vi "Module (Top Level).vi"(8 "error in":errorcluster) -> (0 "error out":errorcluster)   [LabVIEW 2017, in "myPAM.lvlib"]
uses:
  myPAM.lvlib
  MyPAM Controller/Controls/ControlVariables.ctl
  User Events/TypeDefs/Shutdown UE FGV Command.ctl
  Global TypeDefs/Registered Modules.ctl
  Public TypeDefs/Messages.ctl
  Public TypeDefs/Data for Logging.ctl
  MyPAM Controller/Controls/AdmittanceGains.ctl
  <vilib>/Platform/TimedLoop/XDataNode/timing_clust.ctl
  <vilib>/Platform/TimedLoop/XDataNode/nitl_modes.ctl
  <vilib>/Platform/TimedLoop/XDataNode/wakeup.ctl
  Libraries/Real time filter/TypeDefs/Modes.ctl
  Public TypeDefs/Current Position Data.ctl
  <vilib>/FPGAPlugInAG/myRIO-1900/niLvFpga_Open_myRIO-1900.vi
  <vilib>/Utility/error.llb/Error Cluster From Error Code.vi
  <vilib>/rvi/errors/niLvFpgaAdjustHostInterfaceError.vi
  <vilib>/FPGAPlugInAG/myRIO-1900/niLvFpga_Run_myRIO-1900.vi
  <vilib>/FPGAPlugInAG/myRIO-1900/niLvFpga_Close_myRIO-1900.vi
  <vilib>/rvi/interface/nirviOpenFPGA/nirviOpenFPGA.xnode
  <instrlib>/Devantech SRF02/FPGA Example/Serial/Private/FPGA Reference.ctl
  FPGA Bitfiles/myPAM_FPGATarget_FPGA(TopLevel)_Ff4lIePP4-I.lvbitx
  FPGA/FPGA (Top Level).vi
  <vilib>/rvi/interface/nirviReadWriteControl/nirviReadWriteControl.xnode
  <vilib>/rvi/interface/nirviMethod/nirviMethod.xnode
  <vilib>/Platform/TimedLoop/XDataNode/XDataNode.xnode
  <vilib>/rvi/interface/nirviCloseFPGA/nirviCloseFPGA.xnode
  Logger/Logger.lvlib
  Error Handler/Error Handler.lvlib
  Game/Game.lvlib
  <vilib>/Platform/TimedLoop/XDataNode/XDNodeRunTimeDep.lvlib
  WinHost/WinHost.lvlib
  Libraries/Real time filter/RealTimeFilter.lvlib
  NiFpgaLv.dll
  MyPAM Controller/controllerLibrary.lvlib
panel:
  in  "Tragety":dbl
  in  "Tragetx":dbl
  out "output cluster":T1={"ControlFlag"=TRUE, "Fx"=0.0, "Fy"=0.0, "Link1EncPos"=0.0, "Link2EncPos"=0.0, "CurrentX"=0.0, "CurrentY"=0.0, "TargetX"=0.0, "TargetY"=0.0, "DeadZone"=0.0}
  out "U2 2":dbl
  out "U1 2":dbl
  out "PID gains":T2
  out "U2":dbl
  out "U1":dbl
  out "?":cluster{dbl[], dbl[]}(graph)
  out "LINK1_Y_MM":fxp<+/-,34,16> format="%.23g"
  out "LINK1_X_MM":fxp<+/-,34,16> format="%.23g"
  out "LINK2_Y_MM":fxp<+/-,34,16> format="%.23g"
  out "LINK2_X_MM":fxp<+/-,34,16> format="%.23g"
  in  "Control flag":bool=TRUE
  out "LINK1_DEMAND":dbl
  out "LINK2_DEMAND":dbl
  # "mypam"
  # "game"
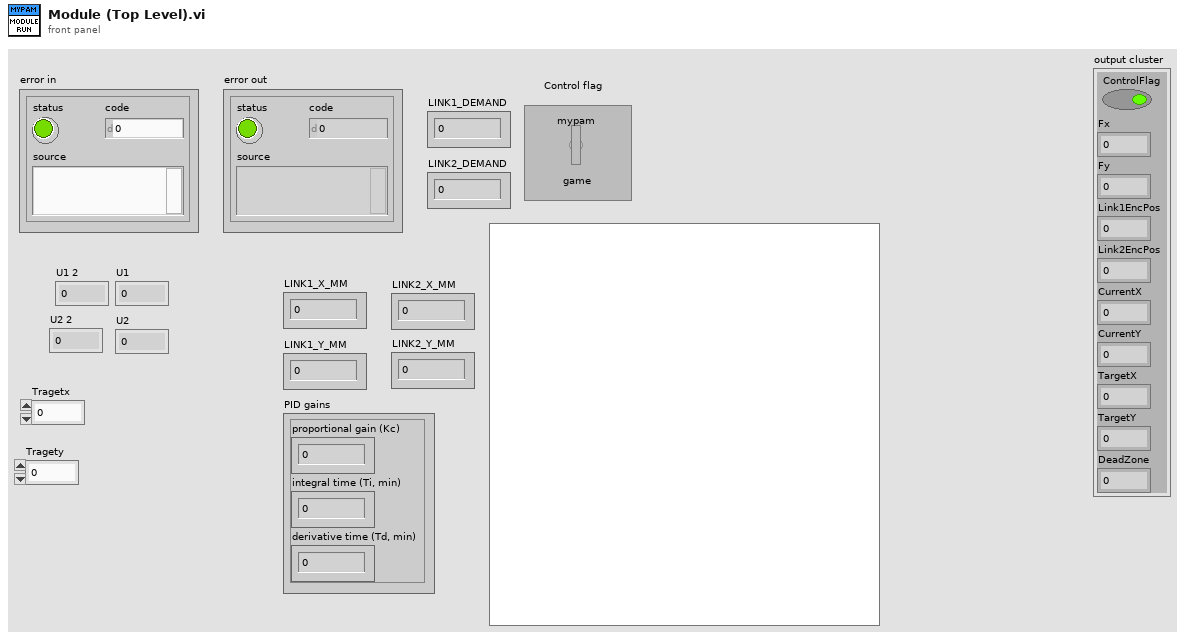
[diagram p1: front panel]
types:
  T1 = typedef "controllerLibrary.lvlib/ControlVariables.ctl" = cluster{"ControlFlag":bool, "Fx":dbl, "Fy":dbl, "Link1EncPos":dbl, "Link2EncPos":dbl, "CurrentX":dbl, "CurrentY":dbl, "TargetX":dbl, "TargetY":dbl, "DeadZone":dbl}
  T2 = cluster{"proportional gain (Kc)":dbl, "integral time (Ti, min)":dbl, "derivative time (Td, min)":dbl}
  T3 = typedef "Registered Modules.ctl" = enum16{"Controller", "DAQ", "Error Handler", "Game", "myPAM", "WinHost", "Logger"}
  T4 = typedef "Shutdown UE FGV Command.ctl" = enum16{"create", "get", "destroy"}
  T5 = typedef "WinHost.lvlib/Module Reference.ctl" = cluster{"calling module":T3, "module queues":T6, "module notifiers":T7}
  T6 = typedef "WinHost.lvlib/Module Queues.ctl" = cluster{"message queue":refnum<queue>, "STM queue":refnum<queue>}
  T7 = typedef "WinHost.lvlib/Module Notifiers.ctl" = cluster{"dummy notifier":refnum<notifier>}
  T8 = typedef "Game.lvlib/Module Reference.ctl" = cluster{"calling module":T3, "module queues":T9, "module notifiers":T10}
  T9 = typedef "Game.lvlib/Module Queues.ctl" = cluster{"message queue":refnum<queue>}
  T10 = typedef "Game.lvlib/Module Notifiers.ctl" = cluster{"dummy notifier":refnum<notifier>}
  T11 = typedef "Logger.lvlib/Module Reference.ctl" = cluster{"calling module":T3, "module queues":T12, "module notifiers":T13}
  T12 = typedef "Logger.lvlib/Module Queues.ctl" = cluster{"message queue":refnum<queue>}
  T13 = typedef "Logger.lvlib/Module Notifiers.ctl" = cluster{"dummy notifier":refnum<notifier>}
  T14 = typedef "myPAM.lvlib/Module Reference.ctl" = cluster{"calling module":T3, "module queues":T15, "module notifiers":T16}
  T15 = typedef "myPAM.lvlib/Module Queues.ctl" = cluster{"message queue":refnum<queue>}
  T16 = typedef "myPAM.lvlib/Module Notifiers.ctl" = cluster{"end eff. pos.":refnum<notifier>}
  T17 = typedef "Error Handler.lvlib/Module Reference.ctl" = cluster{"calling module":T3, "module queues":T18, "module notifiers":T19}
  T18 = typedef "Error Handler.lvlib/Module Queues.ctl" = cluster{"message queue":refnum<queue>}
  T19 = typedef "Error Handler.lvlib/Module Notifiers.ctl" = cluster{"dummy notifier":refnum<notifier>}
  T20 = cluster{"read mode":enum16{"polling", "blocking"}, "write mode":enum16{"polling", "blocking"}}
  T21 = typedef "myPAM.lvlib/Current Position Data.ctl" = cluster{"link 2 x (mm)":dbl, "link 2 y (mm)":dbl, "link 1 x (mm)":dbl, "link 1 y (mm)":dbl}
  T22 = typedef "XDNodeRunTimeDep.lvlib/timing_clust.ctl" = cluster{"Expected End [f-1]":u64, "Actual End [f-1]":u64, "Finished Late? [f-1]":bool, "Expected End [i-1]":u64, "Actual End [i-1]":u64, "Finished Late? [i-1]":bool, "Expected Start [i]":u64, "Actual Start [i]":u64, "Expected Start [f]":u64, "Actual Start [f]":u64, "Source Name":string, "Structure Name":string, "Period":i64, "Deadline":i64, "Offset":i64, "Start":i64, "Priority":i32, "Timeout":i32, "Mode":T23, "Wakeup Reason":T24, "Error":errorcluster, "Source Type":string, "Secondary Source Type":string, "Global End Time":u64, "Global Start Time":u64, "Frame Duration":u64, "Iteration Duration":u64, "Assigned CPU":i32, "I/O Scan Engine Mode":u32}
  T23 = typedef "XDNodeRunTimeDep.lvlib/nitl_modes.ctl" = enum32{"No Change", "Process missed periods, maintain original phase", "Discard missed periods, maintain original phase", "Process missed periods, ignore original phase", "Discard missed periods, ignore original phase"}
  T24 = typedef "XDNodeRunTimeDep.lvlib/wakeup.ctl" = enum32{"Normal", "Aborted", "Asynchronous wakeup", "Timing source error", "Timed loop error", "Timeout"}
  T25 = typedef "FPGA Reference.ctl" = refnum<k20>
  T26 = typedef "myPAM.lvlib/Messages.ctl" = enum16{"calibrate encoders", "enable motors", "disable motors", "operate", "shutdown"}
  T27 = typedef "controllerLibrary.lvlib/AdmittanceGains.ctl" = cluster{"C":dbl, "k":dbl}
  T28 = typedef "myPAM.lvlib/Data for Logging.ctl" = cluster{"end effector x (mm)":dbl, "end effector y (mm)":dbl, "target x (mm)":dbl, "target y (mm)":dbl, "Theta 1":dbl, "Theta 2":dbl, "Omega 1":dbl, "Omega 2":dbl}
  T29 = typedef "myPAM.lvlib/RealTimeFilter.lvlib/Parameters.ctl" = cluster{"number of elements":i32, "start value":dbl, "sinusoidal profile":dbl[], "gaussian profile":dbl[]}
  T30 = typedef "myPAM.lvlib/RealTimeFilter.lvlib/Modes.ctl" = enum16{"Sinusoidal", "Gaussian"}
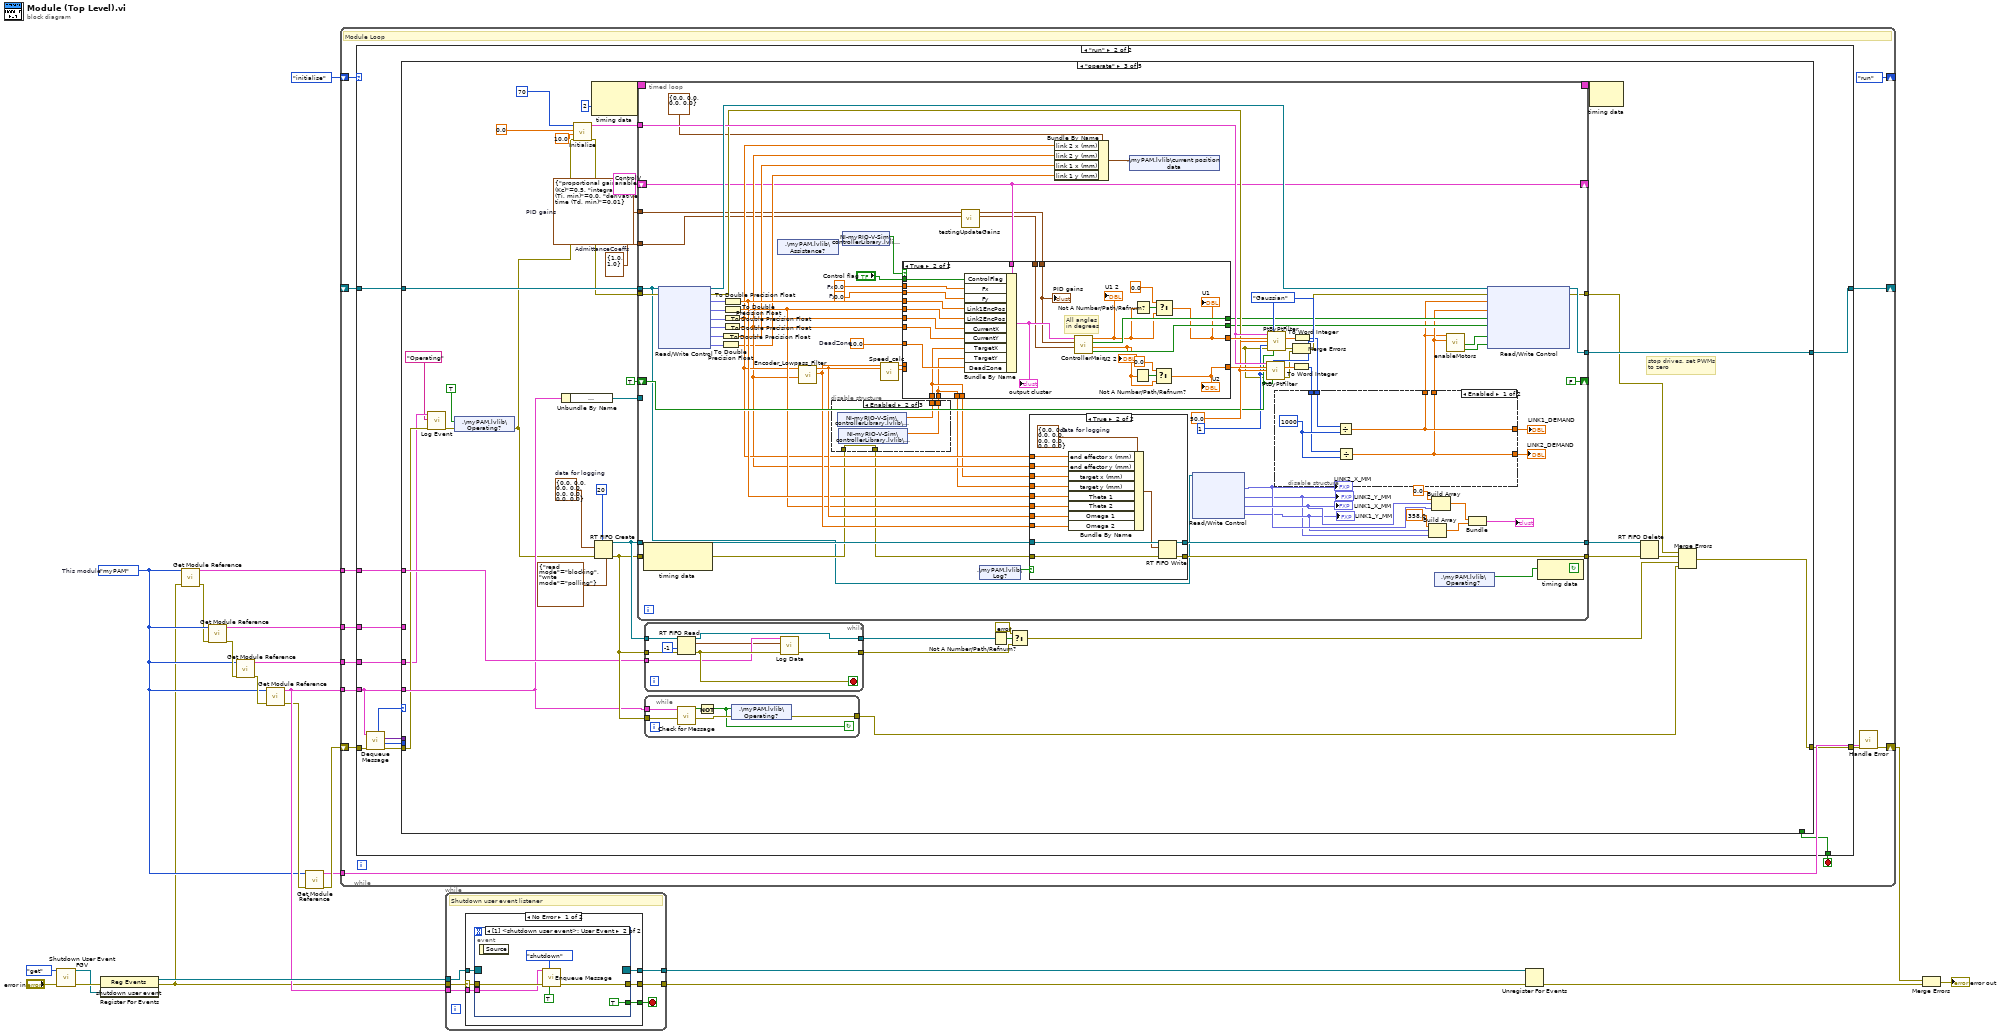
[diagram p0: block diagram]
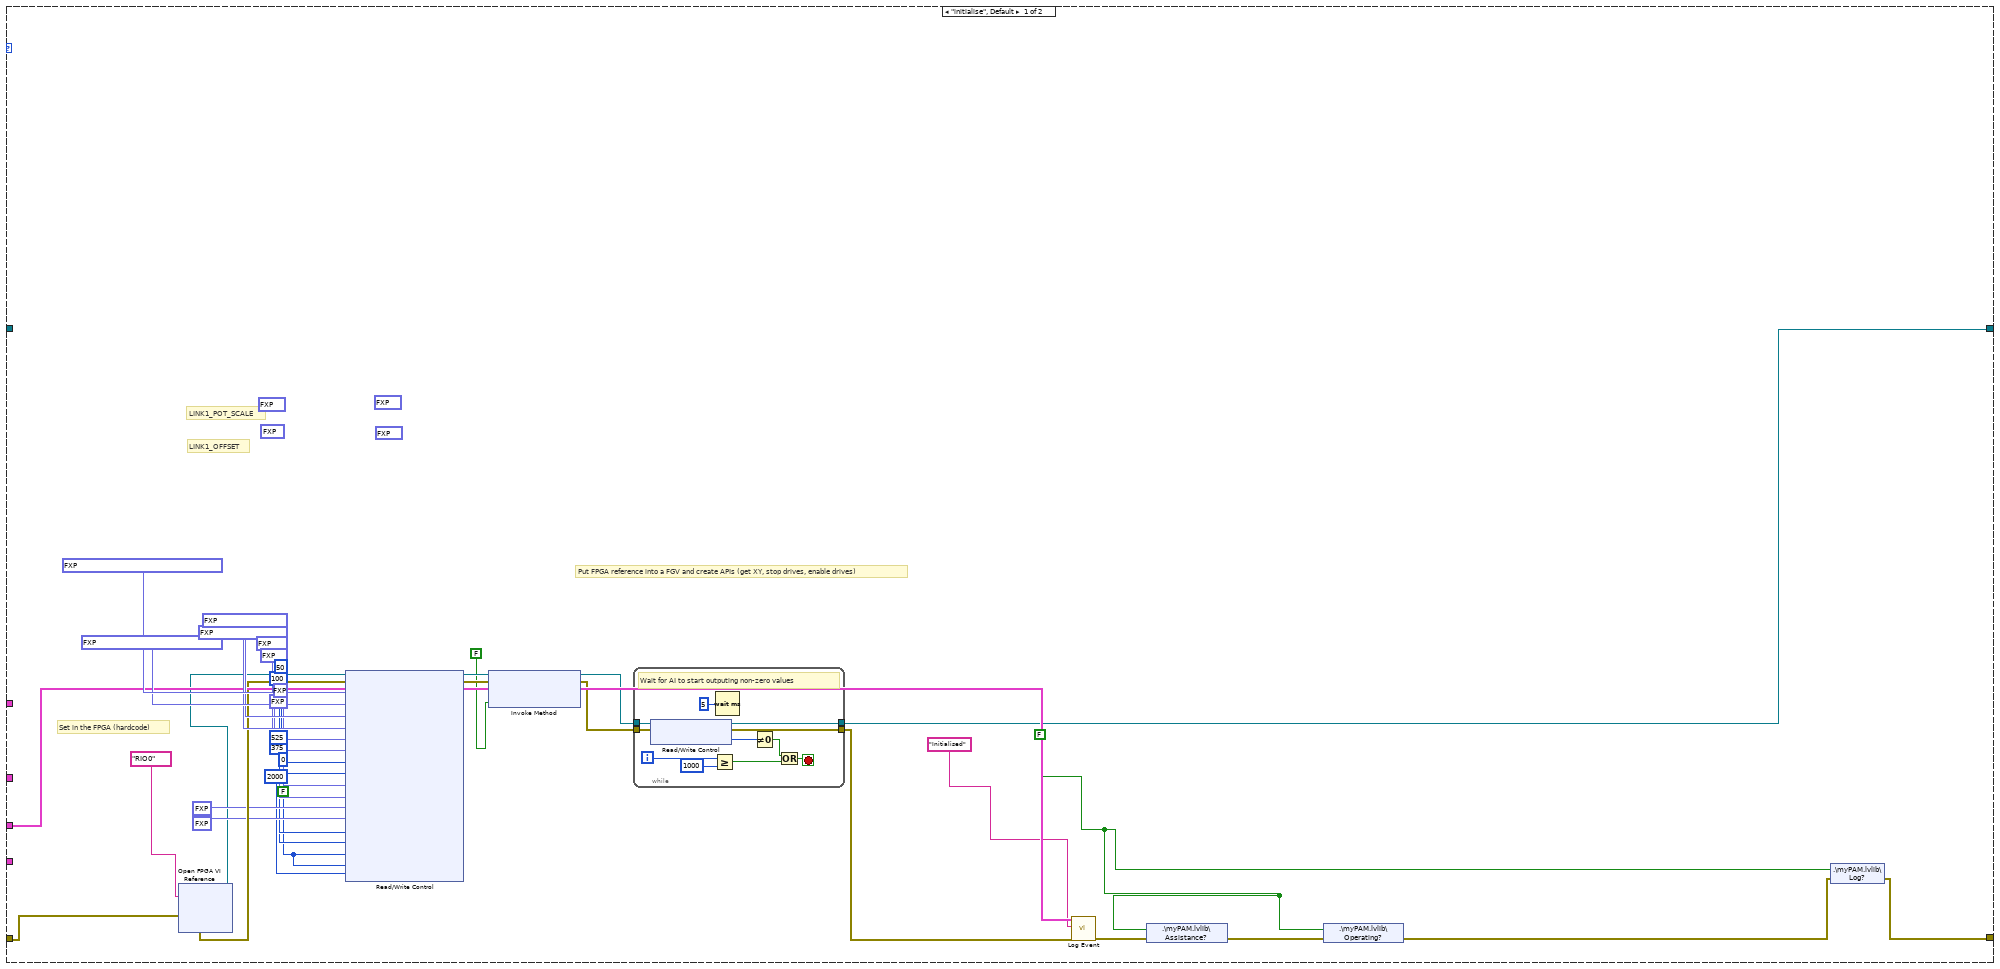
[diagram p2: hidden frame]
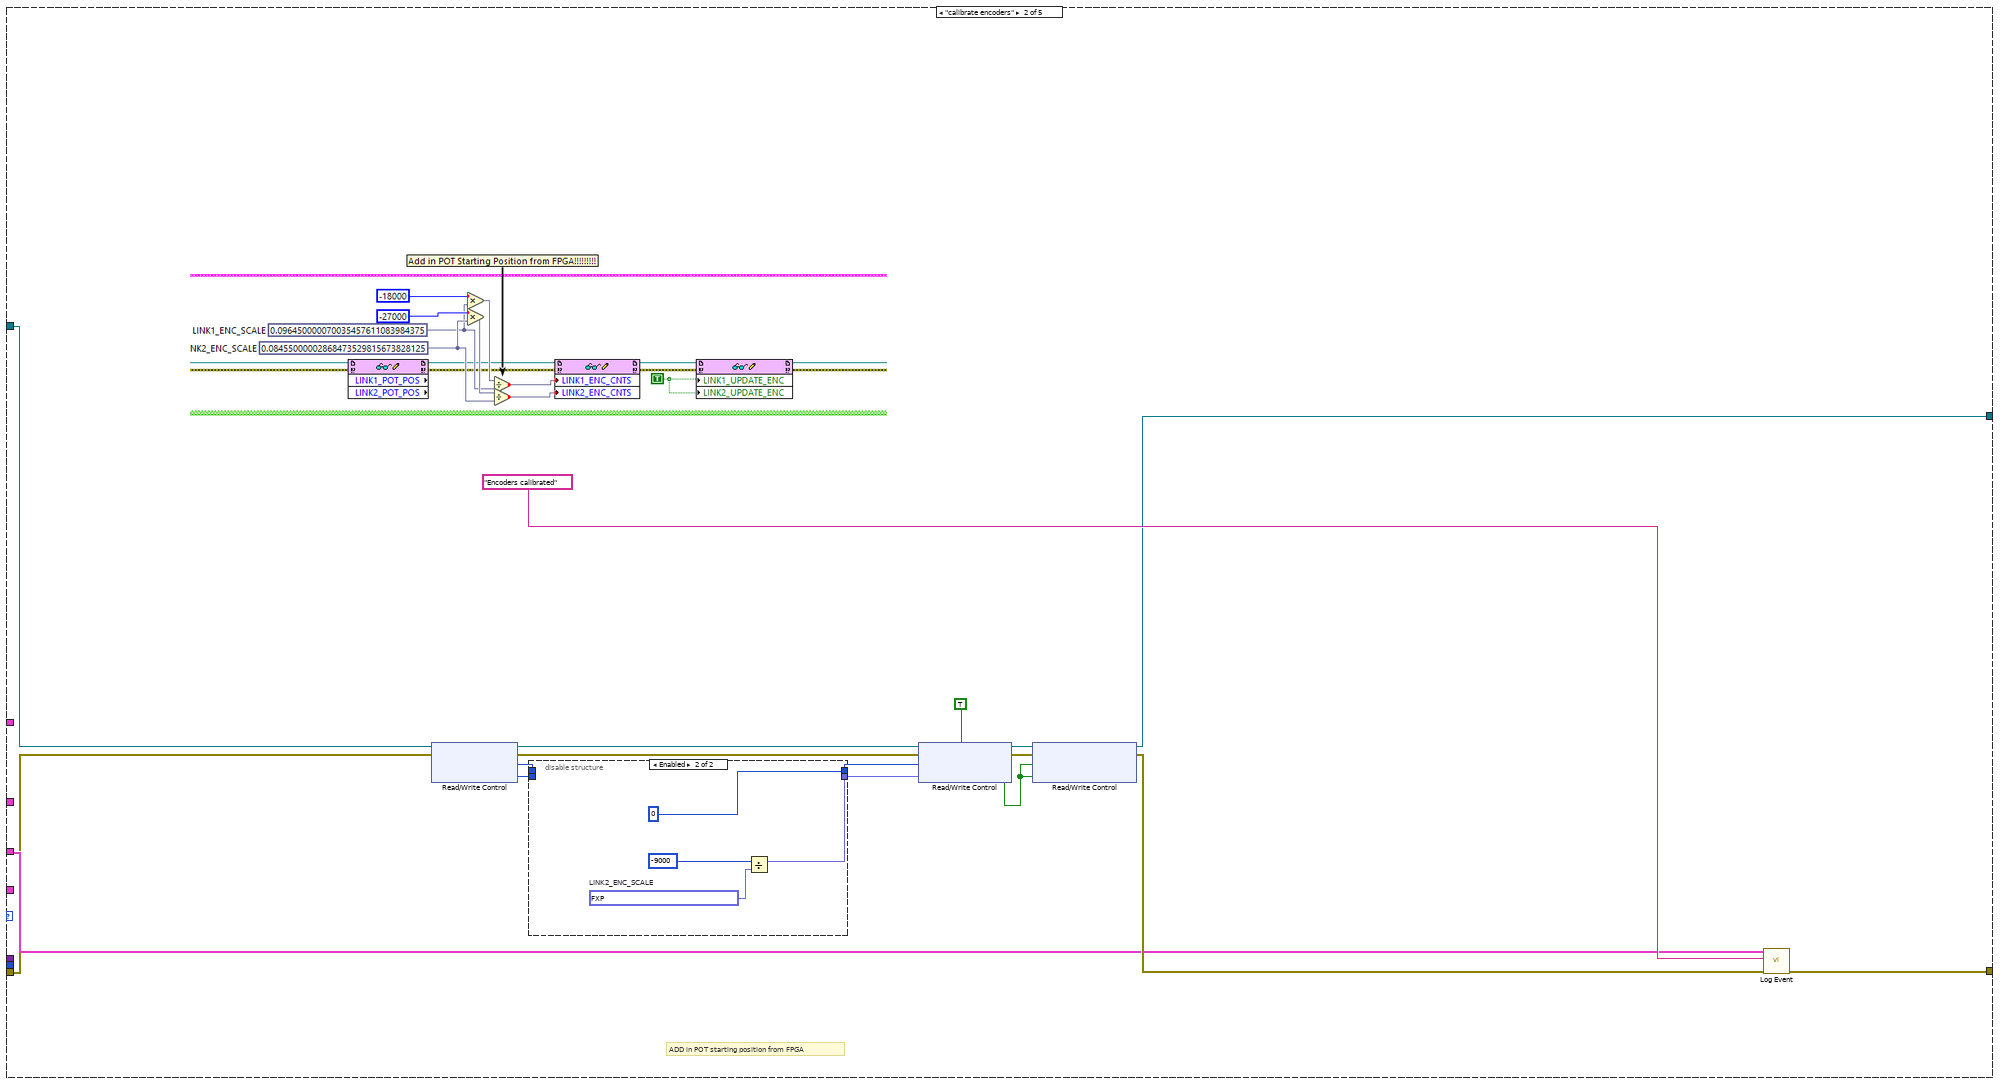
[diagram p4: hidden frame]
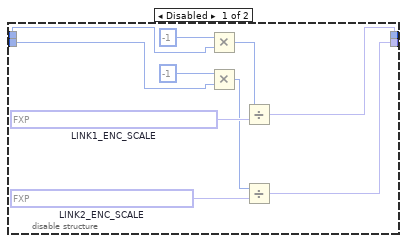
[diagram p5: hidden frame]
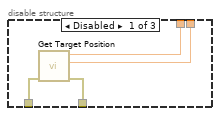
[diagram p6: hidden frame]
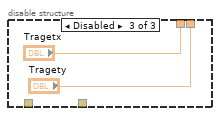
[diagram p7: hidden frame]
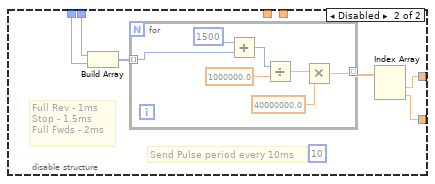
[diagram p8: hidden frame]
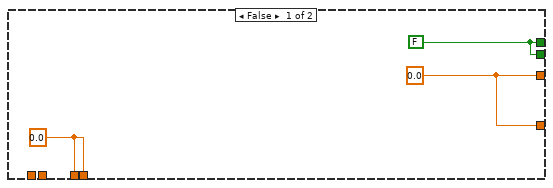
[diagram p9: hidden frame]
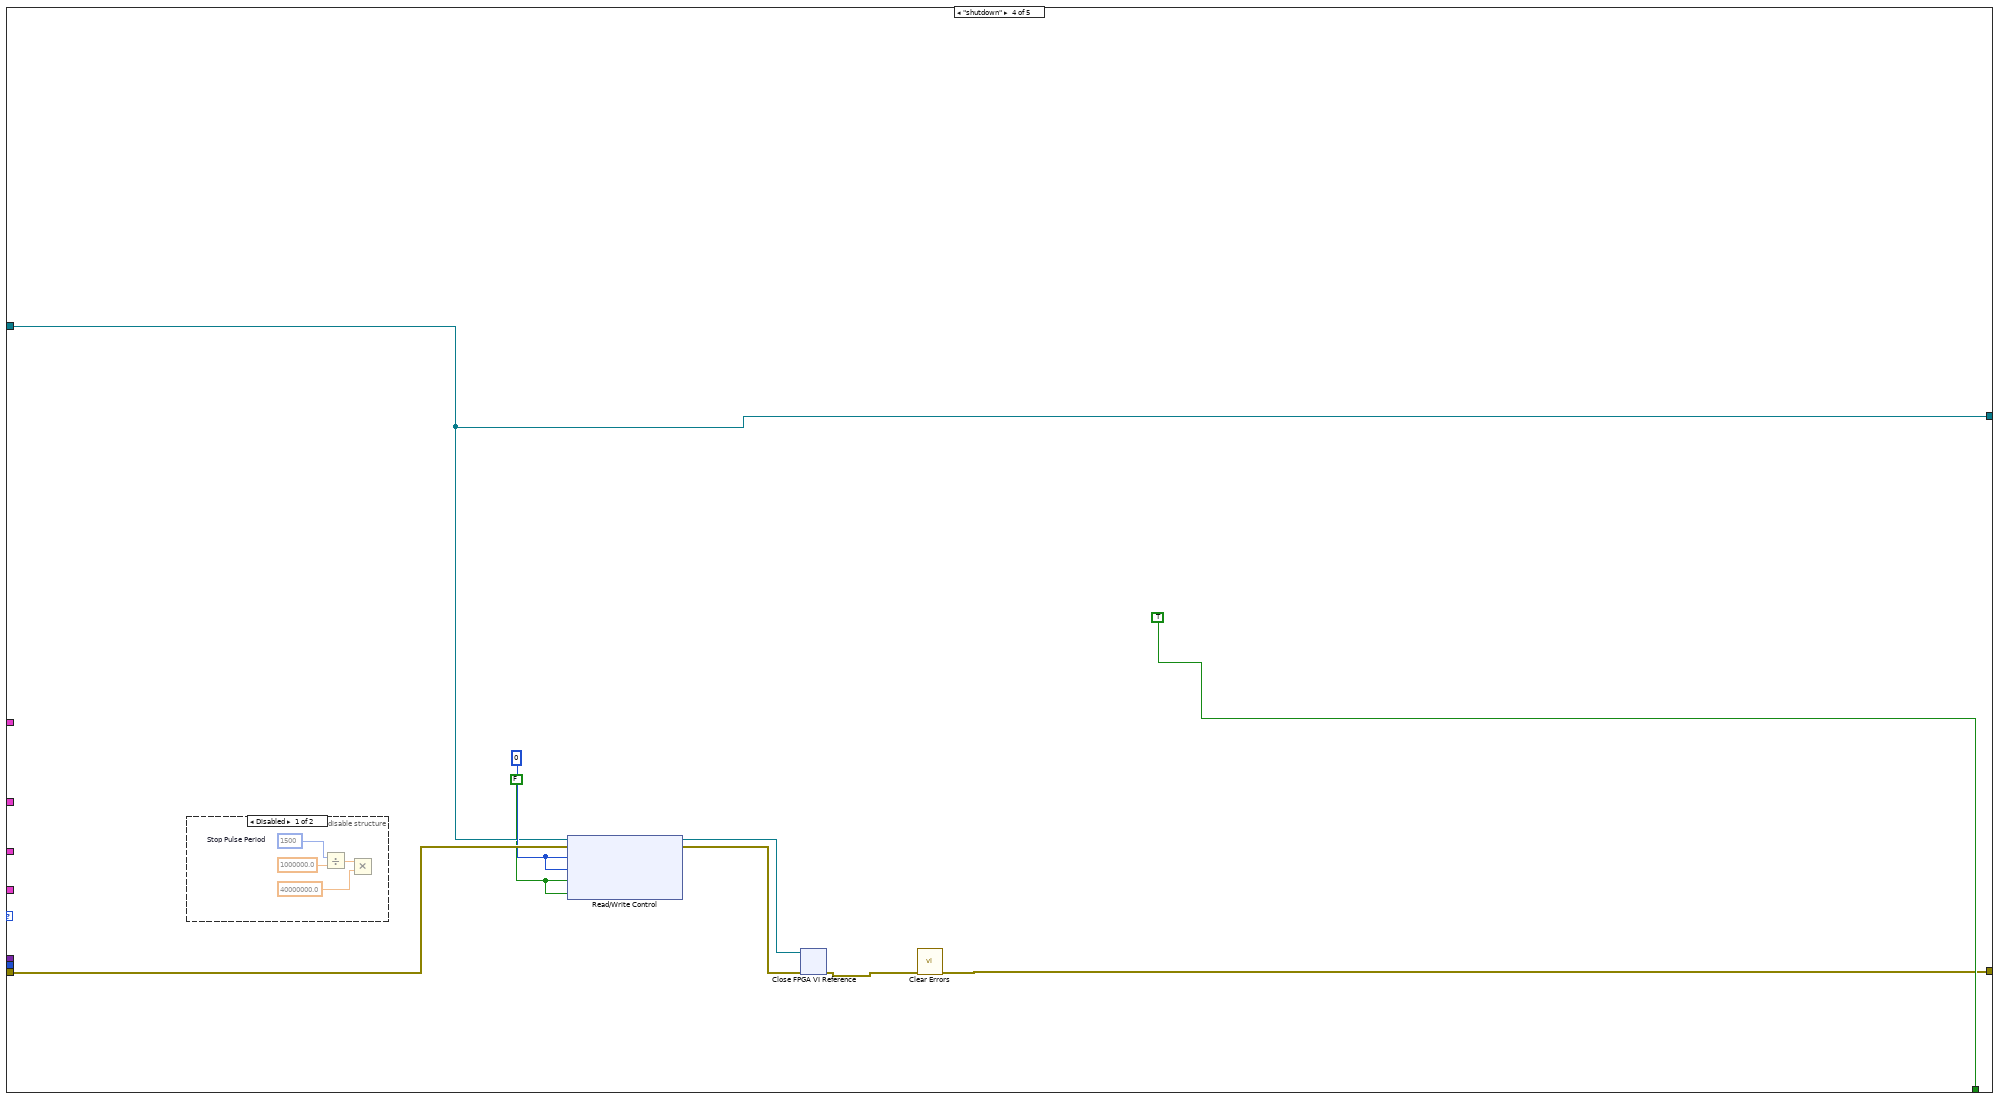
[diagram p11: hidden frame]
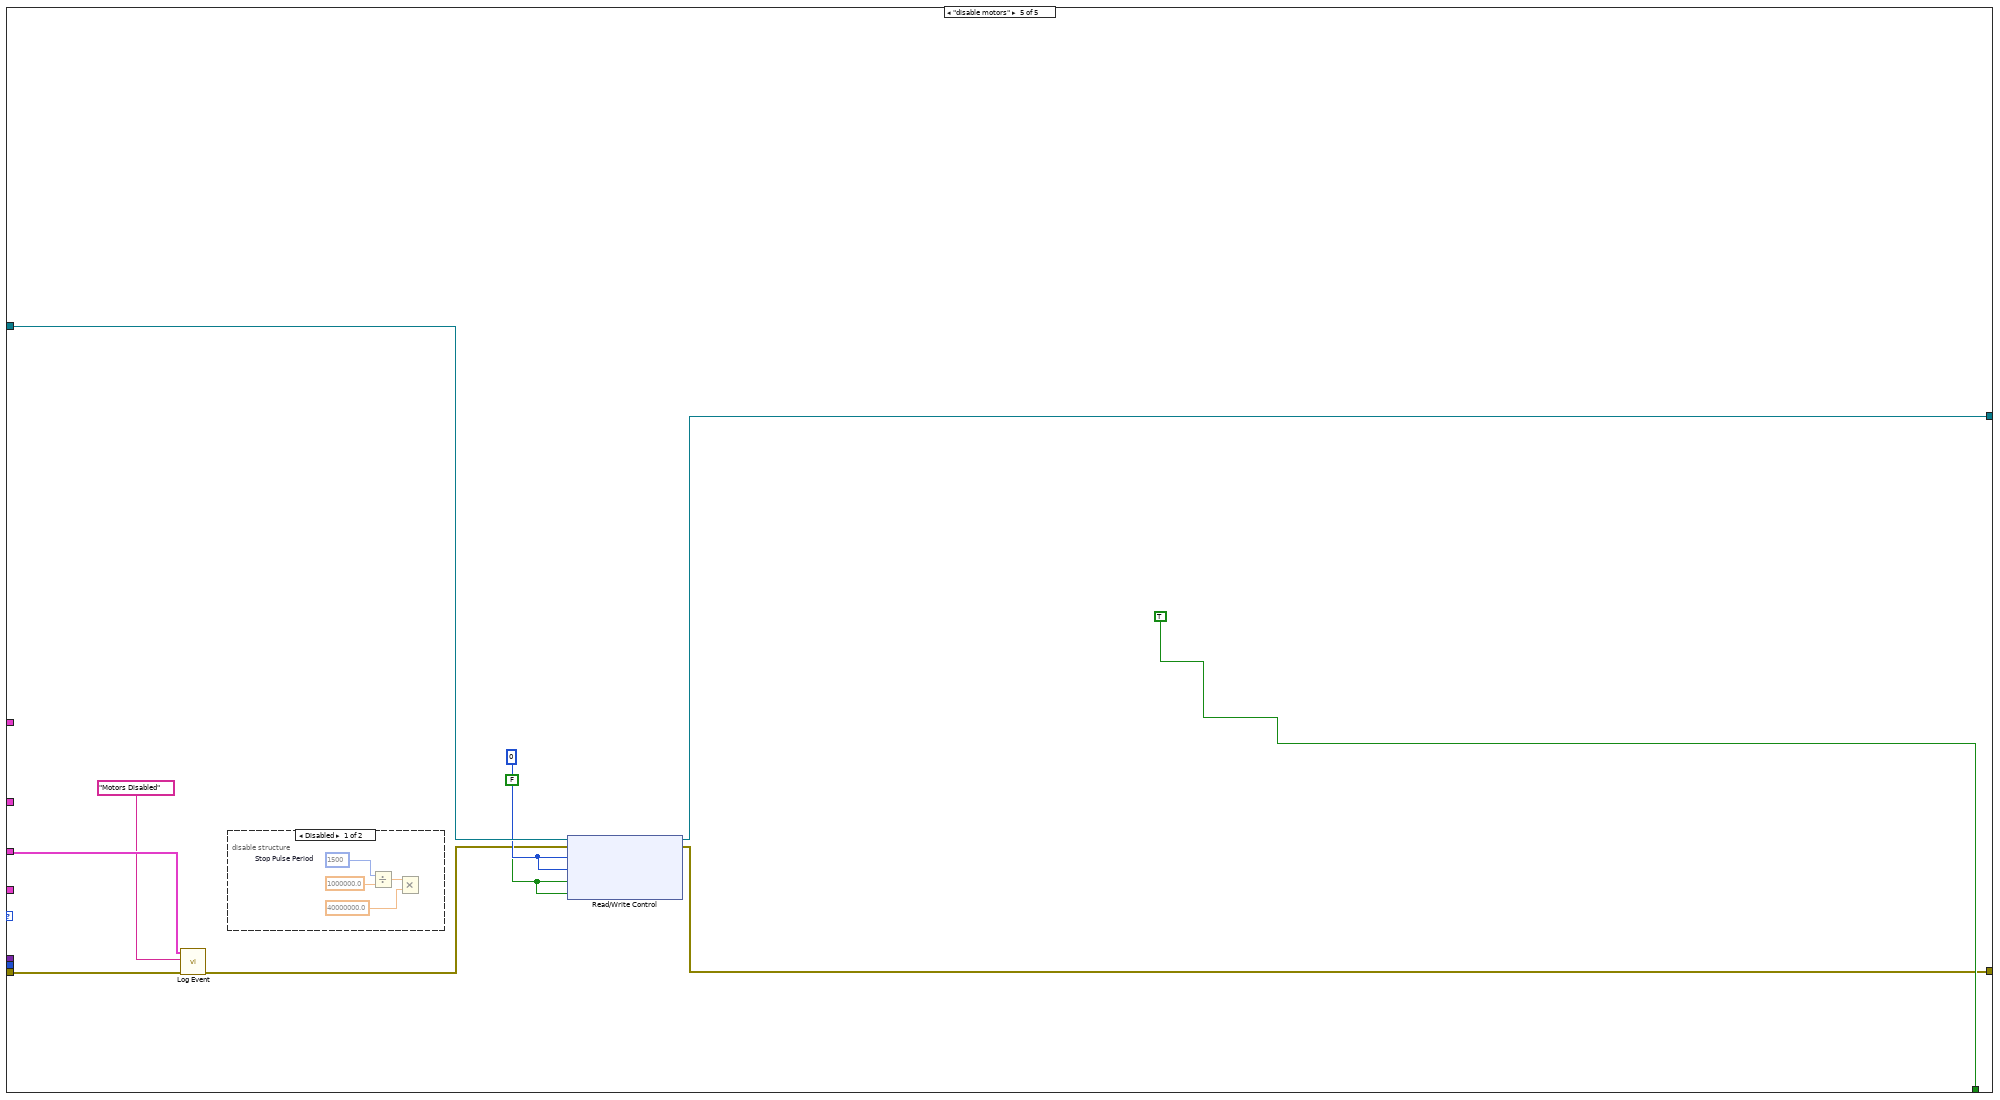
[diagram p13: hidden frame]
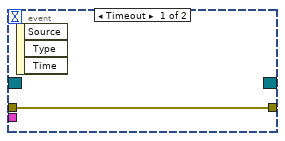
[diagram p15: hidden frame]
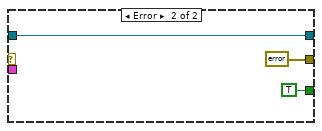
[diagram p16: hidden frame]
diagram:
  w4 = Registered_Modules."myPAM"  # This module
  n1 = call "Shutdown User Event FGV.vi"("error in"="error in", "command"=Shutdown_UE_FGV_Command."get" ("Command")) -> ("error out"=w18:errorcluster, "shutdown user event"=w17:refnum<user-event>)  [unwired: 8 in]
  n2 = register-events(error in=w18, w17) -> (reference out=w22:refnum<event-registration>, error out=w3:errorcluster)  [unwired: 1 in]
  n3 = call "Get Module Reference.vi"("error in"=w3, "calling module"=w4) -> ("error out"=w2:errorcluster, "module reference"=w1:T5)  [unwired: 8 in]
  n4 = call "Get Module Reference.vi"("error in"=w2, "calling module"=w4) -> ("error out"=w8:errorcluster, "module reference"=w5:T8)  [unwired: 8 in]
  n5 = call "Get Module Reference.vi"("error in"=w8, "calling module"=w4) -> ("error out"=w7:errorcluster, "module reference"=w6:T11)  [unwired: 8 in]
  n6 = call "Get Module Reference.vi"("error in"=w7, "calling module"=w4) -> ("error out"=w11:errorcluster, "module reference"=w13:T14)  [unwired: 8 in]
  n7 = call "Get Module Reference.vi"("error in"=w11, "calling module"=w4) -> ("error out"=w10:errorcluster, "module reference"=w9:T17)  [unwired: 8 in]
  n8 = while {
    shift-right: [w29] -> w20
    shift-left: w10 -> [w32]
    tunnel: w13 -> [w36]
    shift-right: [w24] -> _
    shift-left: _ -> [w35]
    shift-right: [enum16{"initialise", "run"}."run"] -> _
    shift-left: enum16{"initialise", "run"}."initialise" -> [w34]
    tunnel: w9 -> [w28]
    tunnel: w6 -> [w27]
    tunnel: w5 -> [w26]
    tunnel: w1 -> [w25]
    stop <- w31 stop-if-true
    # "Module Loop"
    n9 = case shown="\"run\"" w34 {
      tunnel: [w41 w94] -> w30
      tunnel: w36 -> [_ w84]
      tunnel: w35 -> [_ w89]
      tunnel: w32 -> [w56 w87]
      tunnel: [_ w88] -> w31
      tunnel: w27 -> [w62 w86]
      tunnel: w26 -> [_ w85]
      tunnel: w25 -> [_ w83]
      tunnel: [w44 w82] -> w24
      frame "initialise", Default {
        (unwired) FALSE ("Enable Output V")
        (unwired) fxp<+/-,16,16> 15788.0 ("LINK2_OFFSET")
        (unwired) fxp<+/-,32,16> -3352.0 ("LINK2_POT_SCALE")
        (unwired) fxp<+/-,16,16> 5308.0 ("LINK1_OFFSET")
        (unwired) fxp<+/-,32,16> -3396.0 ("LINK1_POT_SCALE")
        w38 = i16 0
        w40 = FALSE ("Enabled?")
        # "LINK1_OFFSET"
        # "LINK1_POT_SCALE"
        # "Set in the FPGA (hardcode)"
        # "Put FPGA reference into a FGV and create APIs (get XY, stop drives, enable drives)"
        n10 = xnode "Open FPGA VI Reference"("error in"=w56, "resource name"=tag "RIO0") -> ("FPGA VI Reference Out"=w55:T25, "error out"=w61:errorcluster)
        n11 = xnode "Read/Write Control"("FPGA VI Reference In"=w55, "error in"=w61, "LINK1_ENC_SCALE"=fxp<+,32,0> 0.21972699998877943, "LINK2_ENC_SCALE"=fxp<+,32,0> 0.12555800005793571, "LINK1_POT_SCALE"=fxp<+/-,32,16> 8.229995727539062, "LINK2_POT_SCALE"=fxp<+/-,32,16> -4.1016998291015625, "LINK1_OFFSET"=fxp<+/-,16,16> -11376.0, "LINK2_OFFSET"=fxp<+/-,16,16> 13125.0, "ENC_DEBOUNCE_CYCLES"=u16 50, "AI_POT_LOOP_US"=u16 100, "X_OFFSET_MM"=fxp<+/-,33,15> 0.0, "Y_OFFSET_MM"=fxp<+/-,33,15> 358.0, "LINK1_LENGTH_MM"=fxp<+,16,12> 358.0, "LINK2_LENGTH_MM"=fxp<+,16,12> 228.0, "LINK1_PWM_MAX"=i16 525, "LINK2_PWM_MAX"=i16 375 ("LINK1_PWM_MAX"), "LINK1_DEMAND_PWM"=w38, "LINK2_DEMAND_PWM"=w38, "PWM Period Loops"=2000) -> ("FPGA VI Reference Out"=w49:T25, "error out"=w50:errorcluster)
        n12 = xnode "Invoke Method"("FPGA VI Reference In"=w49, "error in"=w50, "Wait Until Done (F)"=FALSE) -> ("FPGA VI Reference Out"=w48:T25, "error out"=w47:errorcluster)
        n13 = while {
          tunnel: w48 -> [w81]
          tunnel: w47 -> [w73]
          tunnel: [w72] -> w44
          tunnel: [w71] -> w46
          i -> [w77]
          stop <- w79 stop-if-true
          # "Wait for AI to start outputing non-zero values"
          n14 = xnode "Read/Write Control"("FPGA VI Reference In"=w81, "error in"=w73) -> ("FPGA VI Reference Out"=w72:T25, "error out"=w71:errorcluster, "LINK1_POT_POS"=w80:i32)
          n15 = Greater Or Equal?(x=w77, y=1000) -> (x >= y?=w74:bool)
          n16 = Wait (ms)(milliseconds to wait=u32 5) -> ()  [unwired: 1 out]
          n17 = Not Equal To 0?(x=w80) -> (x != 0?=w78:bool)
          n18 = Or(x=w78, y=w74) -> (x .or. y?=w79:bool)
        }
        n19 = call "Log Event.vi"("error in"=w46, "event"="Initialised" ("string"), "module reference in"=w62) -> ("error out"=w52:errorcluster)  [unwired: 7 in, 1 out]
        n20 = shared-variable ".\\myPAM.lvlib\\Assistance?"(w40, error in=w52) -> (error out=w39:errorcluster)
        n21 = shared-variable ".\\myPAM.lvlib\\Operating?"(w40, error in=w39) -> (error out=w42:errorcluster)
        n22 = shared-variable ".\\myPAM.lvlib\\Log?"(w40, error in=w42) -> (error out=w41:errorcluster)
      }
      frame "run" {
        n23 = call "Dequeue Message.vi"("error in"=w87, "module reference in"=w84) -> ("error out"=w92:errorcluster, "source"=w90:T3, "data"=w91:variant, "message"=w93:T26)  [unwired: 5 in, 1 out]
        n24 = case shown="\"operate\"" w93 {
          tunnel: [w96 w101 w146 w339 w354] -> w94
          tunnel: w92 -> [w96 w99 w142 w337 w350]
          tunnel: w91 -> [_ _ _ _ _]
          tunnel: w90 -> [_ _ _ _ _]
          tunnel: w89 -> [w95 w105 w162 w334 w353]
          tunnel: [_ _ _ TRUE TRUE] -> w88
          tunnel: w86 -> [_ w102 w141 _ w348]
          tunnel: w85 -> [_ _ _ _ _]
          tunnel: w84 -> [_ _ w144 _ _]
          tunnel: [w95 w100 w155 w334 w351] -> w82
          tunnel: w83 -> [_ _ w145 _ _]
          frame Default {
          }
          frame "calibrate encoders" {
            w106 = TRUE
            # "ADD in POT starting position from FPGA"
            n25 = xnode "Read/Write Control"("FPGA VI Reference In"=w105, "error in"=w99) -> ("FPGA VI Reference Out"=w109:T25, "error out"=w110:errorcluster, "LINK1_POT_POS"=w98:i32, "LINK2_POT_POS"=w97:i32)
            n26 = disable-structure shown="Enabled" {
              disable-tunnel: [w122 0] -> w112
              disable-tunnel: [w121 w124] -> w111
              disable-tunnel: w98 -> [w114 _]
              disable-tunnel: w97 -> [w113 _]
              frame Disabled {
                w117 = fxp<+,32,0> 0.12555800005793571  # LINK2_ENC_SCALE
                w118 = fxp<+/-,32,0> 0.21972699998877943  # LINK1_ENC_SCALE
                n27 = Multiply(x=-1, y=w114) -> (x*y=w116:i32)
                n28 = Multiply(x=-1, y=w113) -> (x*y=w115:i32)
                n29 = Divide(x=w116, y=w118) -> (x/y=w122:fxp<+/-,64,65>)
                n30 = Divide(x=w115, y=w117) -> (x/y=w121:fxp<+/-,64,64>)
              }
              frame Enabled {
                w123 = fxp<+,32,0> 0.12555800005793571  # LINK2_ENC_SCALE
                n31 = Divide(x=-9000, y=w123) -> (x/y=w124:fxp<+/-,64,64>)
              }
            }
            n32 = xnode "Read/Write Control"("FPGA VI Reference In"=w109, "error in"=w110, "LINK1_ENC_CNTS"=w112, "LINK2_ENC_CNTS"=w111) -> ("FPGA VI Reference Out"=w108:T25, "error out"=w107:errorcluster)
            n33 = xnode "Read/Write Control"("FPGA VI Reference In"=w108, "error in"=w107, "LINK1_UPDATE_ENC"=w106, "LINK2_UPDATE_ENC"=w106) -> ("FPGA VI Reference Out"=w100:T25, "error out"=w104:errorcluster)
            n34 = call "Log Event.vi"("error in"=w104, "event"="Encoders calibrated", "module reference in"=w102) -> ("error out"=w101:errorcluster)  [unwired: 7 in, 1 out]
          }
          frame "operate" {
            w128 = T2 {"proportional gain (Kc)"=0.5, "integral time (Ti, min)"=0.0, "derivative time (Td, min)"=0.01}  # PID gains
            w127 = T27 {"C"=1.0, "k"=1.0}  # AdmittanceCoeffs
            w159 = T28 {"end effector x (mm)"=0.0, "end effector y (mm)"=0.0, "target x (mm)"=0.0, "target y (mm)"=0.0, "Theta 1"=0.0, "Theta 2"=0.0, "Omega 1"=0.0, "Omega 2"=0.0}  # data for logging
            # "stop drives, set PWMs\nto zero"
            n35 = call "Log Event.vi"("error in"=w142, "event"="Operating", "module reference in"=w141) -> ("error out"=w139:errorcluster)  [unwired: 7 in, 1 out]
            n36 = shared-variable ".\\myPAM.lvlib\\Operating?"(TRUE ("Operating?"), error in=w139) -> (error out=w132:errorcluster)
            n37 = Unbundle By Name(w144) -> ("module notifiers.end eff. pos."=w163:refnum<notifier>)
            n38 = call "Initialise.vi"("error in (no error)"=w132, "gaussian stdev (elements)"=10.0, "start value"=0.0, "number of elements (max 2048)"=70) -> ("error out"=w131:errorcluster, "parameter cluster"=w137:T29)  [unwired: 6 in]
            n39 = node-c288(i64 2 ("Period")) -> (w165:T22)  [unwired: 1 in]
            n40 = RT FIFO Create(1:w159, 3:w132, 4:u32 20 ("size (10)"), 7:T20 {"read mode"=enum."blocking", "write mode"=enum."polling"} ("r/w modes (polling,polling)")) -> (8:w156:refnum<k33>, 11:w150:errorcluster)  [unwired: 4 in, 1 out]
            n41 = timed-loop {
              timing: w165 -> [_]
              timing-out: [_] -> w164
              tunnel: w162 -> [w180]
              tunnel: w163 -> [_]
              tunnel: w150 -> [w191]
              tunnel: w156 -> [w240]
              tunnel: [w239] -> w158
              tunnel: [w238] -> w157
              tunnel: [w232] -> w155
              tunnel: w131 -> [w237]
              tunnel: w137 -> [w226]
              shift-right: [FALSE] -> _
              shift-left: TRUE -> [w222]
              tunnel: [w216] -> w130
              shift-right: [w188] -> _
              shift-left: T1 {"ControlFlag"=TRUE, "Fx"=0.0, "Fy"=0.0, "Link1EncPos"=0.0, "Link2EncPos"=0.0, "CurrentX"=0.0, "CurrentY"=0.0, "TargetX"=0.0, "TargetY"=0.0, "DeadZone"=0.0} -> [w188]
              tunnel: w128 -> [w182]
              tunnel: w127 -> [w181]
              stop <- w242 continue-if-true
              w189 = 10.0  # DeadZone
              w194 = 0.0  # Fy
              w195 = 0.0  # Fx
              w221 = i64 1 ("dt")
              w225 = 50.0 ("max speed")
              w223 = Modes."Gaussian" ("Mode")
              # "From host"
              n42 = node-c288() -> ()  [unwired: 1 in, 2 out]
              n43 = xnode "Read/Write Control"("FPGA VI Reference In"=w180, "error in"=w237) -> ("FPGA VI Reference Out"=w231:T25, "error out"=w220:errorcluster, "Angle 1 (deg)"=w234:fxp<+/-,15,10>, "Angle 2 (deg)"=w233:fxp<+/-,15,10>, "LINK2_X_MM"=w236:fxp<+/-,34,16>, "LINK2_Y_MM"=w235:fxp<+/-,34,16>, "LINK1_X_MM"=w213:fxp<+/-,34,16>, "LINK1_Y_MM"=w212:fxp<+/-,34,16>)
              n44 = To Double Precision Float(number=w213) -> (double precision float=w197:dbl)
              n45 = To Double Precision Float(number=w212) -> (double precision float=w196:dbl)
              n46 = To Double Precision Float(number=w236) -> (double precision float=w199:dbl)
              n47 = To Double Precision Float(number=w235) -> (double precision float=w198:dbl)
              n48 = To Double Precision Float(number=w234) -> (double precision float=w201:dbl)
              n49 = To Double Precision Float(number=w233) -> (double precision float=w200:dbl)
              n50 = shared-variable ".\\myPAM.lvlib\\Assistance?"() -> ()  [unwired: 1 in, 2 out]
              n51 = call "Encoder_Lowpass_Filter.vi"("LINK2_ENC_POS"=w198, "LINK1_ENC_POS"=w199) -> ("LINK2_ENC_POS_FILTERED"=w205:dbl, "LINK1_ENC_POS_FILTERED"=w206:dbl)  [unwired: 6 in]
              n52 = disable-structure shown="Enabled" {
                disable-tunnel: [w246 w248 "Tragetx"] -> w193
                disable-tunnel: [w245 w247 "Tragety"] -> w192
                disable-tunnel: w191 -> [w244 w249 _]
                disable-tunnel: [w243 w249 _] -> w190
                frame Disabled {
                  n53 = call "Get Target Position.vi"("error in"=w244) -> ("error out"=w243:errorcluster, "target y (mm)"=w245:dbl, "target x (mm)"=w246:dbl)  [unwired: 8 in]
                }
                frame Enabled {
                  n54 = shared-variable "NI-myRIO-V-Sim\\controllerLibrary.lvlib\\testingtargetX"() -> (w248:dbl)  [unwired: 1 in, 1 out]
                  n55 = shared-variable "NI-myRIO-V-Sim\\controllerLibrary.lvlib\\testingtargetY"() -> (w247:dbl)  [unwired: 1 in, 1 out]
                }
                frame Disabled {
                }
              }
              n56 = shared-variable "NI-myRIO-V-Sim\\controllerLibrary.lvlib\\testing"() -> (w170:bool)  [unwired: 1 in, 1 out]
              n57 = call "Speed_calc.vi"("X"=w206, "Y"=w205) -> ("Vy"=w202:dbl, "Vx"=w203:dbl)  [unwired: 8 in]
              n58 = call "testingUpdateGains.vi"("AdmittanceCoeffs"=w181, "PID gains"=w182) -> ("AdmittanceCoeffs"=w184:T27, "PID gains"=w183:T2)  [unwired: 8 in]
              n59 = case shown="True" w170 {
                tunnel: [w272 w278] -> w230
                tunnel: [w272 w273] -> w228
                tunnel: [w271 w284] -> w207
                tunnel: "Control flag" -> [_ w295]
                tunnel: w203 -> [_ _]
                tunnel: w202 -> [_ _]
                tunnel: w201 -> [_ w292]
                tunnel: w200 -> [_ w291]
                tunnel: w199 -> [_ w290]
                tunnel: w198 -> [_ w289]
                tunnel: w195 -> [_ w294]
                tunnel: w194 -> [_ w293]
                tunnel: w193 -> [_ w282]
                tunnel: w192 -> [_ w281]
                tunnel: w188 -> [_ w296]
                tunnel: w189 -> [_ w288]
                tunnel: w183 -> [_ w286]
                tunnel: w184 -> [_ w285]
                tunnel: [w271 w283] -> w187
                tunnel: [w270 w282] -> w186
                tunnel: [w270 w281] -> w185
                frame False {
                  w270 = 0.0
                  w271 = FALSE
                  w272 = 0.0
                }
                frame True {
                  # "All angles\nin degrees"
                  n60 = Bundle By Name(cluster=w296, "ControlFlag"=w295, "Fx"=w294, "Fy"=w293, "Link1EncPos"=w292, "Link2EncPos"=w291, "CurrentX"=w290, "CurrentY"=w289, "TargetX"=w282, "TargetY"=w281, "DeadZone"=w288) -> (w287:T1)
                  "output cluster" <- w287
                  n61 = call "ControllerMain.vi"("AdmittanceCoeffs"=w285, "PID gains"=w286, 11:w287) -> ("Direction 2"=w283:bool, "U2"=w274:dbl, "Direction1"=w284:bool, "U1"=w279:dbl)  [unwired: 5 in]
                  "U1 2" <- w279
                  "U2 2" <- w274
                  n62 = Not A Number/Path/Refnum?(number/path/refnum=w274) -> (NaN/Path/Refnum?=w275:bool)
                  n63 = Not A Number/Path/Refnum?(number/path/refnum=w279) -> (NaN/Path/Refnum?=w280:bool)
                  n64 = Select(t=0.0, s=w275, f=w274) -> (s? t:f=w273:dbl)
                  "U2" <- w273
                  n65 = Select(t=0.0, s=w280, f=w279) -> (s? t:f=w278:dbl)
                  "U1" <- w278
                  "PID gains" <- w286
                }
              }
              n66 = shared-variable ".\\myPAM.lvlib\\Log?"() -> (w241:bool)  [unwired: 1 in, 1 out]
              n67 = case shown="True" w241 {
                tunnel: w199 -> [_ w312]
                tunnel: w198 -> [_ w311]
                tunnel: w240 -> [w298 w309]
                tunnel: w190 -> [w297 w308]
                tunnel: [w298 w306] -> w239
                tunnel: [w297 w305] -> w238
                tunnel: w201 -> [_ w304]
                tunnel: w200 -> [_ w303]
                tunnel: w206 -> [_ w302]
                tunnel: w205 -> [_ w301]
                tunnel: w186 -> [_ w300]
                tunnel: w185 -> [_ w299]
                frame False {
                }
                frame True {
                  w310 = T28 {"end effector x (mm)"=0.0, "end effector y (mm)"=0.0, "target x (mm)"=0.0, "target y (mm)"=0.0, "Theta 1"=0.0, "Theta 2"=0.0, "Omega 1"=0.0, "Omega 2"=0.0}  # data for logging
                  n68 = Bundle By Name(cluster=w310, "end effector x (mm)"=w312, "end effector y (mm)"=w311, "target x (mm)"=w300, "target y (mm)"=w299, "Theta 1"=w304, "Theta 2"=w303, "Omega 1"=w302, "Omega 2"=w301) -> (w307:T28)
                  n69 = RT FIFO Write(0:w309, 1:w307, 3:w308) -> (8:w306:refnum<k33>, 11:w305:errorcluster)  [unwired: 2 in, 2 out]
                }
              }
              n70 = Bundle By Name(cluster=T21 {"link 2 x (mm)"=0.0, "link 2 y (mm)"=0.0, "link 1 x (mm)"=0.0, "link 1 y (mm)"=0.0} ("current position data"), "link 2 x (mm)"=w199, "link 2 y (mm)"=w198, "link 1 x (mm)"=w197, "link 1 y (mm)"=w196) -> (w214:T21)
              n71 = shared-variable ".\\myPAM.lvlib\\current position data"(w214) -> ()  [unwired: 1 in, 1 out]
              n72 = xnode "Read/Write Control"("FPGA VI Reference In"=w180) -> ("LINK2_X_MM"=w174:fxp<+/-,34,16>, "LINK2_Y_MM"=w172:fxp<+/-,34,16>, "LINK1_X_MM"=w175:fxp<+/-,34,16>, "LINK1_Y_MM"=w173:fxp<+/-,34,16>)  [unwired: 1 in, 2 out]
              "LINK2_X_MM" <- w174
              "LINK2_Y_MM" <- w172
              "LINK1_X_MM" <- w175
              "LINK1_Y_MM" <- w173
              n73 = call "PtByPtFilter.vi"("parameter cluster"=w226, "Mode"=w223, "demand"=w228, "max speed"=w225, "dt"=w221, "error in"=w220, "reset"=w222) -> ("filtered signal"=w227:dbl, "error out"=w218:errorcluster)  [unwired: 7 in]
              n74 = call "PtByPtFilter.vi"("parameter cluster"=w226, "Mode"=w223, "demand"=w230, "max speed"=w225, "dt"=w221, "error in"=w220, "reset"=w222) -> ("filtered signal"=w229:dbl, "error out"=w219:errorcluster)  [unwired: 7 in]
              n75 = To Word Integer(number=w227) -> (16bit integer=w210:i16)
              n76 = Merge Errors(w219, w218) -> (w217:errorcluster)
              n77 = To Word Integer(number=w229) -> (16bit integer=w211:i16)
              n78 = disable-structure shown="Enabled" {
                disable-tunnel: w211 -> [w255 w262]
                disable-tunnel: w210 -> [w254 w261]
                disable-tunnel: [w253 w258] -> w209
                disable-tunnel: [w252 w257] -> w208
                disable-tunnel: [w253 _] -> w168
                disable-tunnel: [w252 _] -> w169
                frame Enabled {
                  w256 = i16 1000 ("y")
                  n79 = Divide(x=w255, y=w256) -> (x/y=w253:dbl)
                  n80 = Divide(x=w254, y=w256) -> (x/y=w252:dbl)
                }
                frame Disabled {
                  (unwired) u16 10 ("Pulse 1 Wait (ms)")
                  # "Full Rev - 1ms\nStop - 1.5ms\nFull Fwds - 2ms"
                  # "Send Pulse period every 10ms"
                  n81 = Build Array(w262, w261) -> (w260:i16[])
                  n82 = for {
                    tunnel: w260 -> [w266] mode=indexing
                    tunnel: [w267] -> w259 mode=indexing
                    n83 = Add(x=i16 1500 ("y"), y=w266) -> (x+y=w265:i16)
                    n84 = Divide(x=w265, y=1000000.0) -> (x/y=w263:dbl)
                    n85 = Multiply(x=w263, y=40000000.0) -> (x*y=w267:dbl)
                  }
                  n86 = Index Array(array=w259) -> (element #1=w258:dbl, element #2=w257:dbl)  [unwired: 2 in]
                }
              }
              "LINK2_DEMAND" <- w208
              "LINK1_DEMAND" <- w209
              n87 = Build Array(358.0 ("element"), w173, w172) -> (w176:dbl[])
              n88 = Build Array(0.0 ("element"), w175, w174) -> (w177:dbl[])
              n89 = shared-variable ".\\myPAM.lvlib\\Operating?"() -> (w242:bool)  [unwired: 1 in, 1 out]
              n90 = call "enableMotors.vi"("Link 2 Demand"=w169, "Link 1 Demand"=w168) -> ("Enable motor 2"=w166:bool, "Enable motor 1"=w167:bool)  [unwired: 6 in, 2 out]
              n91 = Bundle(w177, w176) -> (→"?":cluster{dbl[], dbl[]})  [unwired: 1 in]
              n92 = xnode "Read/Write Control"("FPGA VI Reference In"=w231, "error in"=w217, "Link_1 Duty"=w168, "Link_2 Duty"=w169, "LINK1_DRIVE_ENABLED"=w207, "LINK2_DRIVE_ENABLED"=w187, "Enable motor 1"=w167, "Enable motor 2"=w166) -> ("FPGA VI Reference Out"=w232:T25, "error out"=w216:errorcluster)
              n93 = node-c288() -> ()  [unwired: 1 in, 1 out]
            }
            n94 = while {
              tunnel: w156 -> [w332]
              tunnel: w150 -> [w331]
              tunnel: [w326] -> w154
              tunnel: [w327] -> w152
              tunnel: w145 -> [w328]
              stop <- w329 stop-if-true
              n95 = RT FIFO Read(0:w332, 2:-1 ("timeout in ms (0)"), 3:w331) -> (8:w326:refnum<k33>, 9:w325:T28, 11:w329:errorcluster)  [unwired: 1 in, 2 out]
              n96 = call "Log Data.vi"("error in"=w329, "data for logging"=w325, "module reference in"=w328) -> ("error out"=w327:errorcluster)  [unwired: 7 in, 1 out]
            }
            n97 = while {
              tunnel: w144 -> [w324]
              tunnel: w150 -> [w323]
              tunnel: [w319] -> w147
              stop <- w320 continue-if-true
              n98 = call "Check for Message.vi"("error in"=w323, "module reference"=w324) -> ("error out"=w321:errorcluster, "new element available"=w322:bool)  [unwired: 8 in]
              n99 = Not(x=w322) -> (.not. x?=w320:bool)
              n100 = shared-variable ".\\myPAM.lvlib\\Operating?"(w320, error in=w321) -> (error out=w319:errorcluster)
            }
            n101 = Not A Number/Path/Refnum?(number/path/refnum=w154) -> (NaN/Path/Refnum?=w153:bool)
            n102 = Select(t=errorcluster {"status"=FALSE, "code"=0, "source"=""}, s=w153, f=w152) -> (s? t:f=w148:errorcluster)
            n103 = node-c288(w164) -> ()  [unwired: 1 out]
            n104 = RT FIFO Delete(0:w158, 3:w157) -> (11:w149:errorcluster)  [unwired: 1 in]
            n105 = Merge Errors(w130, w149, w148, w147) -> (w146:errorcluster)
          }
          frame "shutdown" {
            w333 = FALSE
            w335 = i16 0 ("LINK1_DEMAND_PWM")
            n106 = disable-structure shown="Disabled" {
              frame Disabled {
                w342 = i16 1500  # Stop Pulse Period
                n107 = Divide(x=w342, y=1000000.0) -> (x/y=w344:dbl)
                n108 = Multiply(x=w344, y=40000000.0) -> ()  [unwired: 1 out]
              }
              frame Enabled {
              }
            }
            n109 = xnode "Read/Write Control"("FPGA VI Reference In"=w334, "error in"=w337, "LINK1_DEMAND_PWM"=w335, "LINK2_DEMAND_PWM"=w335, "LINK1_DRIVE_ENABLED"=w333, "LINK2_DRIVE_ENABLED"=w333) -> ("FPGA VI Reference Out"=w336:T25, "error out"=w338:errorcluster)
            n110 = xnode "Close FPGA VI Reference"("FPGA VI Reference In"=w336, "error in"=w338) -> ("error out"=w341:errorcluster)
            n111 = call <vilib>:"Clear Errors.vi"("error in (no error)"=w341) -> ("error out"=w339:errorcluster)  [unwired: 5 in, 1 out]
          }
          frame "disable motors" {
            w346 = FALSE
            w352 = i16 0 ("LINK1_DEMAND_PWM")
            n112 = call "Log Event.vi"("error in"=w350, "event"="Motors Disabled", "module reference in"=w348) -> ("error out"=w349:errorcluster)  [unwired: 7 in, 1 out]
            n113 = disable-structure shown="Disabled" {
              frame Disabled {
                w356 = i16 1500  # Stop Pulse Period
                n114 = Divide(x=w356, y=1000000.0) -> (x/y=w358:dbl)
                n115 = Multiply(x=w358, y=40000000.0) -> ()  [unwired: 1 out]
              }
              frame Enabled {
              }
            }
            n116 = xnode "Read/Write Control"("FPGA VI Reference In"=w353, "error in"=w349, "LINK1_DEMAND_PWM"=w352, "LINK2_DEMAND_PWM"=w352, "LINK1_DRIVE_ENABLED"=w346, "LINK2_DRIVE_ENABLED"=w346) -> ("FPGA VI Reference Out"=w351:T25, "error out"=w354:errorcluster)
          }
        }
      }
    }
    n117 = call "Handle Error.vi"("module reference in"=w28, "error in"=w30) -> ("error out"=w29:errorcluster)  [unwired: 9 in]
  }
  n118 = while {
    tunnel: w22 -> [w365]
    tunnel: [w364] -> w21
    tunnel: w3 -> [w362]
    tunnel: [w361] -> w15
    tunnel: w13 -> [w360]
    stop <- w363 stop-if-true
    # "Shutdown user event listener"
    n119 = case shown="No Error" w362 {
      selector: w362 -> [w368 _]
      tunnel: w365 -> [w371 w380]
      tunnel: [w370 w380] -> w364
      tunnel: [w369 TRUE] -> w363
      tunnel: [w367 errorcluster {"status"=FALSE, "code"=0, "source"=""} ("error out")] -> w361
      tunnel: w360 -> [w366 _]
      frame No Error {
        n120 = event shown="[1] <shutdown user event>: User Event" {
          selector: w371 -> [_ _]
          dyn-events: [_ _] -> w370
          timeout: _ -> [_ _]
          tunnel: w368 -> [w372 w376]
          tunnel: [w372 w375] -> w367
          tunnel: [_ TRUE] -> w369
          tunnel: w366 -> [_ w374]
          event Timeout {
            n121 = event-data() -> ()  [unwired: 1 in, 3 out]
          }
          event User Event {
            n122 = event-data() -> ()  [unwired: 1 in, 1 out]
            n123 = call "Enqueue Message.vi"("high priority"=TRUE, "message"=Messages."shutdown", "error in"=w376, "module reference in"=w374) -> ("error out"=w375:errorcluster)  [unwired: 6 in, 1 out]
          }
        }
      }
      frame Error {
      }
    }
  }
  n124 = Unregister For Events(event registration refnum=w21, error in=w15) -> (error out=w16:errorcluster)
  n125 = Merge Errors(w20, w16) -> (→"error out":errorcluster)
